vi "numeric_const_type_adapter.vi"() -> ()   [LabVIEW 2023]
panel:
  in  "Numeric 4":dbl
  in  "Numeric 3":i32
  out "Numeric 2":dbl=32.0
  out "Numeric":i32=21
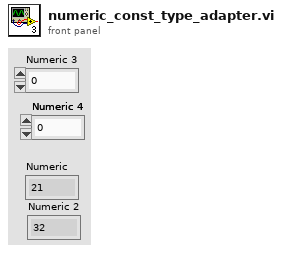
[diagram p1: front panel]
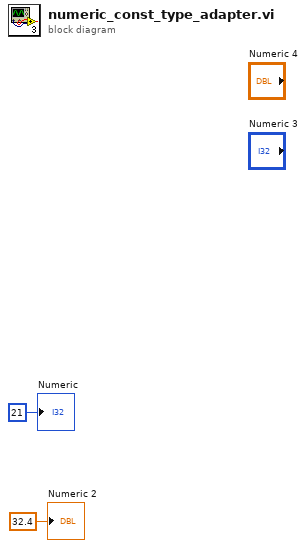
[diagram p0: block diagram]
diagram:
  "Numeric" <- 21
  "Numeric 2" <- 32.4
